vi "2_5.vi"() -> ()   [LabVIEW 2010]
panel:
  out "Numeric 2":i32
  in  "Numeric":i32
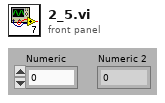
[diagram p1: front panel]
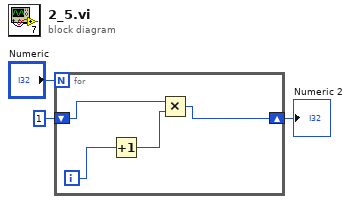
[diagram p0: block diagram]
diagram:
  n1 = for {
    N: "Numeric" -> [_]
    shift-right: [w4] -> w1
    shift-left: 1 -> [w5]
    i -> [w6]
    n2 = Increment(x=w6) -> (x+1=w7:i32)
    n3 = Multiply(x=w5, y=w7) -> (x*y=w4:i32)
  }
  "Numeric 2" <- w1
